vi "TCF Data to  Measurement Description.vi"(8 "error in (no error)":errorcluster, 11 "NI Generic Parser in":refnum<class "NI Generic Parser.lvclass">=refnum) -> (0 "error out":errorcluster, 2 "Measurements Out":T1[](array[typedef]), 3 "NI Generic Parser out":refnum<class "NI Generic Parser.lvclass">)   [LabVIEW 2018, in "NI Generic Parser.lvlib" / "NI Generic Parser.lvclass"]
uses:
  NI Generic Parser.lvclass
  Plugins/Measurement Data.lvlibp/Measurement Data.lvclass
  Plugins/File Parsing Interface.lvlibp/Controls/Parsed Measurement.ctl
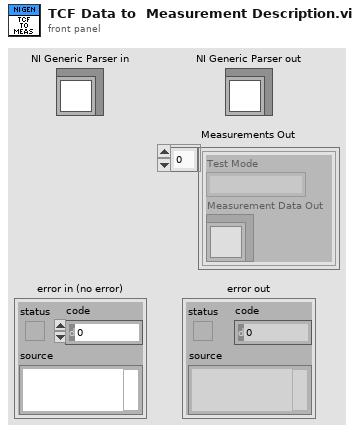
[diagram p1: front panel]
types:
  T1 = typedef "File Parsing Interface.lvlibp/File Parsing Interface.lvclass/Parsed Measurement.ctl" = cluster{"Test Mode":string, "Measurement Data Out":refnum<class "Measurement Data.lvclass">}
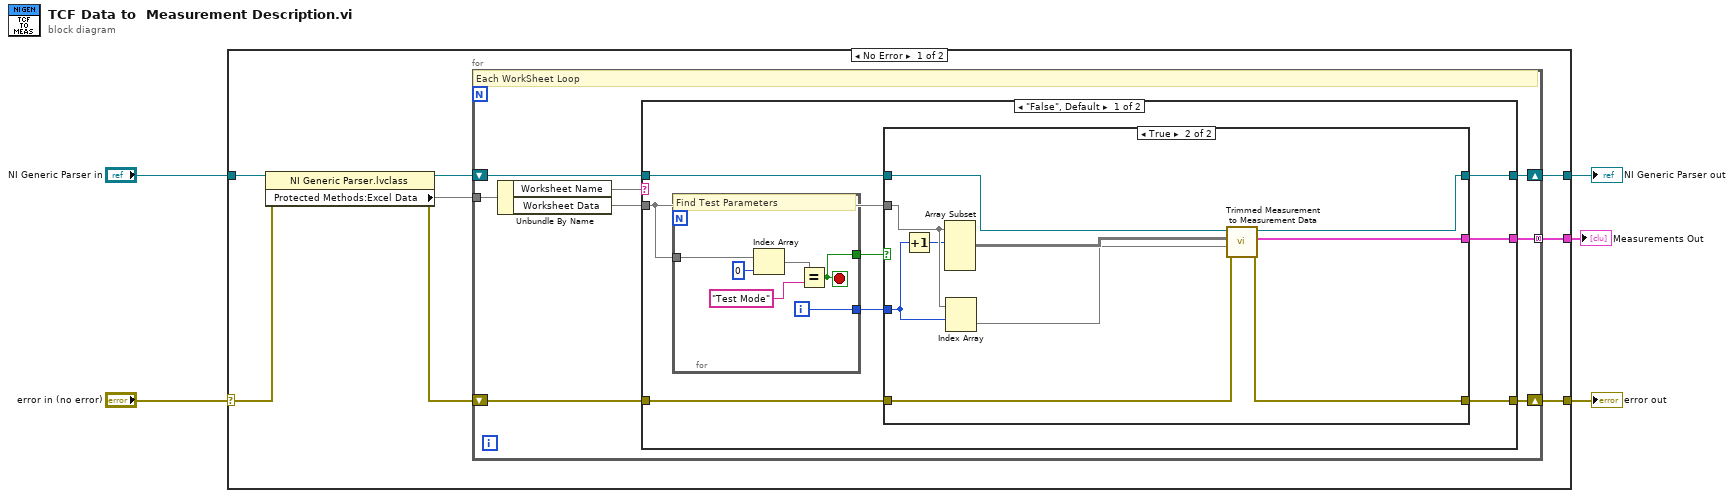
[diagram p0: block diagram]
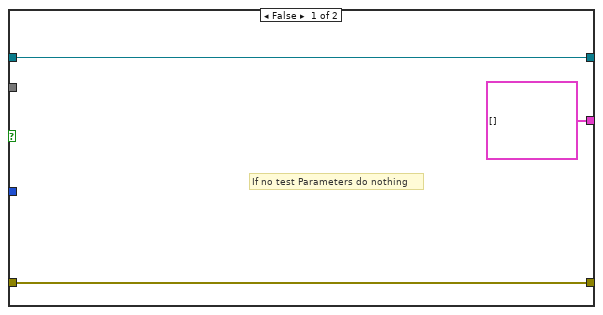
[diagram p2: hidden frame]
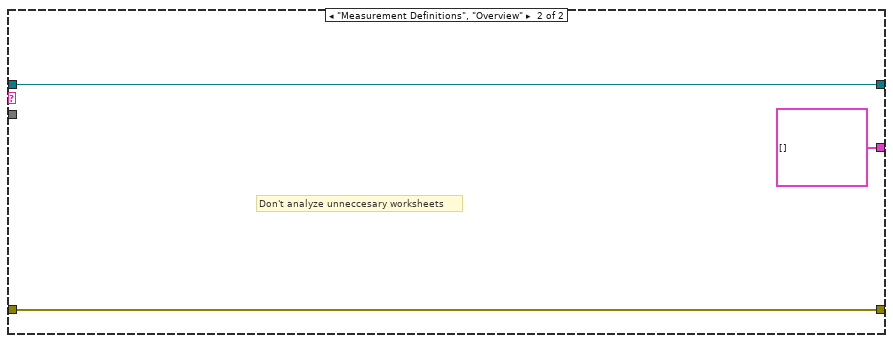
[diagram p3: hidden frame]
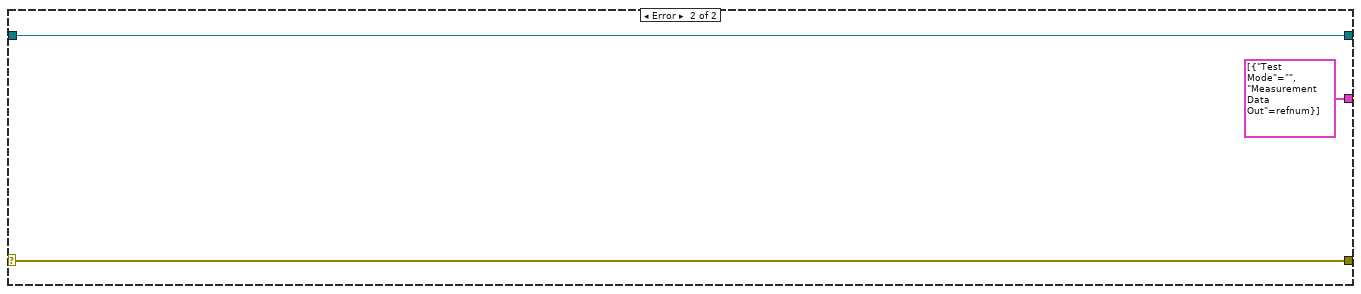
[diagram p4: hidden frame]
diagram:
  n1 = case shown="No Error" "error in (no error)" {
    selector: "error in (no error)" -> [w13 w54]
    tunnel: [w10 w54] -> w4
    tunnel: [w8 w53] -> w1
    tunnel: "NI Generic Parser in" -> [w12 w53]
    tunnel: [w6 T1[] [{"Test Mode"="", "Measurement Data Out"=refnum}] ("MEasurements From Work Sheet")] -> w2
    frame No Error {
      n2 = property class="NI Generic Parser.lvclass"(reference=w12, error in=w13) -> (reference out=w7:refnum<class "NI Generic Parser.lvclass">, error out=w11:errorcluster, "Protected Methods:Excel Data"=w9)
      n3 = for {
        shift-right: [w20] -> w10
        shift-left: w11 -> [w21]
        tunnel: w9 -> [w19]
        shift-right: [w16] -> w8
        shift-left: w7 -> [w15]
        tunnel: [w14] -> w6 mode=concatenating
        # "Each WorkSheet Loop"
        n4 = Unbundle By Name(w19) -> ("Worksheet Name"=w18, "Worksheet Data"=w17)
        n5 = case shown="\"False\", Default" w18 {
          tunnel: w21 -> [w24 w51]
          tunnel: [w23 w51] -> w20
          tunnel: w17 -> [w28 _]
          tunnel: [w25 w50] -> w16
          tunnel: w15 -> [w26 w50]
          tunnel: [w22 T1[] [] ("MEasurements From Work Sheet")] -> w14
          frame "False", Default {
            n6 = for {
              tunnel: w28 -> [w48]
              tunnel: [w44] -> w27
              tunnel: [w43] -> w29
              i -> [w44]
              stop <- w43 stop-if-true
              # "Find Test Parameters"
              n7 = Index Array(array=w48, index=0) -> (element=w46)
              n8 = Equal?(x=w46, y="Test Mode") -> (x = y?=w43:bool)
            }
            n9 = case shown="True" w29 {
              tunnel: w28 -> [_ w42]
              tunnel: w27 -> [_ w33]
              tunnel: w26 -> [w32 w39]
              tunnel: [w32 w38] -> w25
              tunnel: w24 -> [w31 w36]
              tunnel: [w31 w35] -> w23
              tunnel: [T1[] [] ("MEasurements From Work Sheet") w37] -> w22
              frame False {
                # "If no test Parameters do nothing"
              }
              frame True {
                n10 = Increment(x=w33) -> (x+1=w34:i32)
                n11 = Array Subset(array=w42, index (row)=w34) -> (w41:void[][])  [unwired: 3 in]
                n12 = Index Array(array=w42, index (row)=w33) -> (element=w40)  [unwired: 1 in]
                n13 = call "Trimmed Measurement to Measurement Data.vi"("Error In"=w36, "Measurement Keys"=w40, "Trimmed Worksheet Data"=w41, "NI Generic Parser in"=w39) -> ("Error Out"=w35:errorcluster, "Measurements From Work Sheet"=w37:T1[], "NI Generic Parser out"=w38:refnum<class "NI Generic Parser.lvclass">)  [unwired: 5 in]
              }
            }
          }
          frame "Measurement Definitions", "Overview" {
            # "Don't analyze unneccesary worksheets"
          }
        }
      }
    }
    frame Error {
    }
  }
  "error out" <- w4
  "NI Generic Parser out" <- w1
  "Measurements Out" <- w2
